vi "Merce Cmd.vi"() -> ()   [LabVIEW 2009]
panel:
  out "output Header":string[](array[string])
  out "Array":string[][](array[string])
  out "AMP":string[](array[string])
  out "FT":string[](array[string])
  out "RT":string[](array[string])
  out "WS1050 Cmd":string[](array[string])
  out "WS1050 Name":string[](array[string])
  in  "WS1050 C1L Cmd":string[](array[string])=["074101", "074100", "074102", "074100", "074104", "074108", "07410C", "074110", "074114", "074118", "07411C", "074120", "074124", "074128", "07412C", "074130", "074134", "074138", "074139", "07413B", "074139", "074138", "074134", "074130", "07412C", "074128", "074124", "074120", "07411C", "074118", "074114", "074110", "07410C", "074108", "074104", "074100", "", "", "", "", "", "", "", "", "", "", "", "", "", "", "", "", "", "", "", "", "", "", "", "", "", "", "", "", "", "", "", "", "", "", "", ""]
  in  "C1L":string[](array[string])=["C1L_S0F1_ON", "C1L_S0F1_OFF", "C1L_S0F2_ON", "C1L_S0F2_OFF", "C1L_S1_UP", "C1L_S2_UP", "C1L_S3_UP", "C1L_S4_UP", "C1L_S5_UP", "C1L_S6_UP", "C1L_S7_UP", "C1L_S8_UP", "C1L_S9_UP", "C1L_S10_UP", "C1L_S11_UP", "C1L_S12_UP", "C1L_S13_UP", "C1L_S14_UP", "C1L_S14F1_UP", "C1L_S14F12_UP", "C1L_S14F1_DN", "C1L_S14_DN", "C1L_S13_DN", "C1L_S12_DN", "C1L_S11_DN", "C1L_S10_DN", "C1L_S9_DN", "C1L_S8_DN", "C1L_S7_DN", "C1L_S6_DN", "C1L_S5_DN", "C1L_S4_DN", "C1L_S3_DN", "C1L_S2_DN", "C1L_S1_DN", "C1L_ALL_OFF"]
  in  "C3L":string[](array[string])=["C3L_S0F1_ON", "C3L_S0F1_OFF", "C3L_S0F2_ON", "C3L_S0F2_OFF", "C3L_S1_UP", "C3L_S2_UP", "C3L_S3_UP", "C3L_S4_UP", "C3L_S5_UP", "C3L_S6_UP", "C3L_S7_UP", "C3L_S8_UP", "C3L_S9_UP", "C3L_S10_UP", "C3L_S11_UP", "C3L_S12_UP", "C3L_S13_UP", "C3L_S14_UP", "C3L_S14F1_UP", "C3L_S14F12_UP", "C3L_S14F1_DN", "C3L_S14_DN", "C3L_S13_DN", "C3L_S12_DN", "C3L_S11_DN", "C3L_S10_DN", "C3L_S9_DN", "C3L_S8_DN", "C3L_S7_DN", "C3L_S6_DN", "C3L_S5_DN", "C3L_S4_DN", "C3L_S3_DN", "C3L_S2_DN", "C3L_S1_DN", "C3L_ALL_OFF"]
  in  "C2L":string[](array[string])=["C2L_S0F1_ON", "C2L_S0F1_OFF", "C2L_S0F2_ON", "C2L_S0F2_OFF", "C2L_S1_UP", "C2L_S2_UP", "C2L_S3_UP", "C2L_S4_UP", "C2L_S5_UP", "C2L_S6_UP", "C2L_S7_UP", "C2L_S8_UP", "C2L_S9_UP", "C2L_S10_UP", "C2L_S11_UP", "C2L_S12_UP", "C2L_S13_UP", "C2L_S14_UP", "C2L_S14F1_UP", "C2L_S14F12_UP", "C2L_S14F1_DN", "C2L_S14_DN", "C2L_S13_DN", "C2L_S12_DN", "C2L_S11_DN", "C2L_S10_DN", "C2L_S9_DN", "C2L_S8_DN", "C2L_S7_DN", "C2L_S6_DN", "C2L_S5_DN", "C2L_S4_DN", "C2L_S3_DN", "C2L_S2_DN", "C2L_S1_DN", "C2L_ALL_OFF"]
  in  "WS1050 C3L Cmd":string[](array[string])=["074301", "074300", "074302", "074300", "074304", "074308", "07430C", "074310", "074314", "074318", "07431C", "074320", "074324", "074328", "07432C", "074330", "074334", "074338", "074339", "07433B", "074339", "074338", "074334", "074330", "07432C", "074328", "074324", "074320", "07431C", "074318", "074314", "074310", "07430C", "074308", "074304", "074300"]
  in  "WS1050 C2L Cmd":string[](array[string])=["074201", "074200", "074202", "074200", "074204", "074208", "07420C", "074210", "074214", "074218", "07421C", "074220", "074224", "074228", "07422C", "074230", "074234", "074238", "074239", "07423B", "074239", "074238", "074234", "074230", "07422C", "074228", "074224", "074220", "07421C", "074218", "074214", "074210", "07420C", "074208", "074204", "074200"]
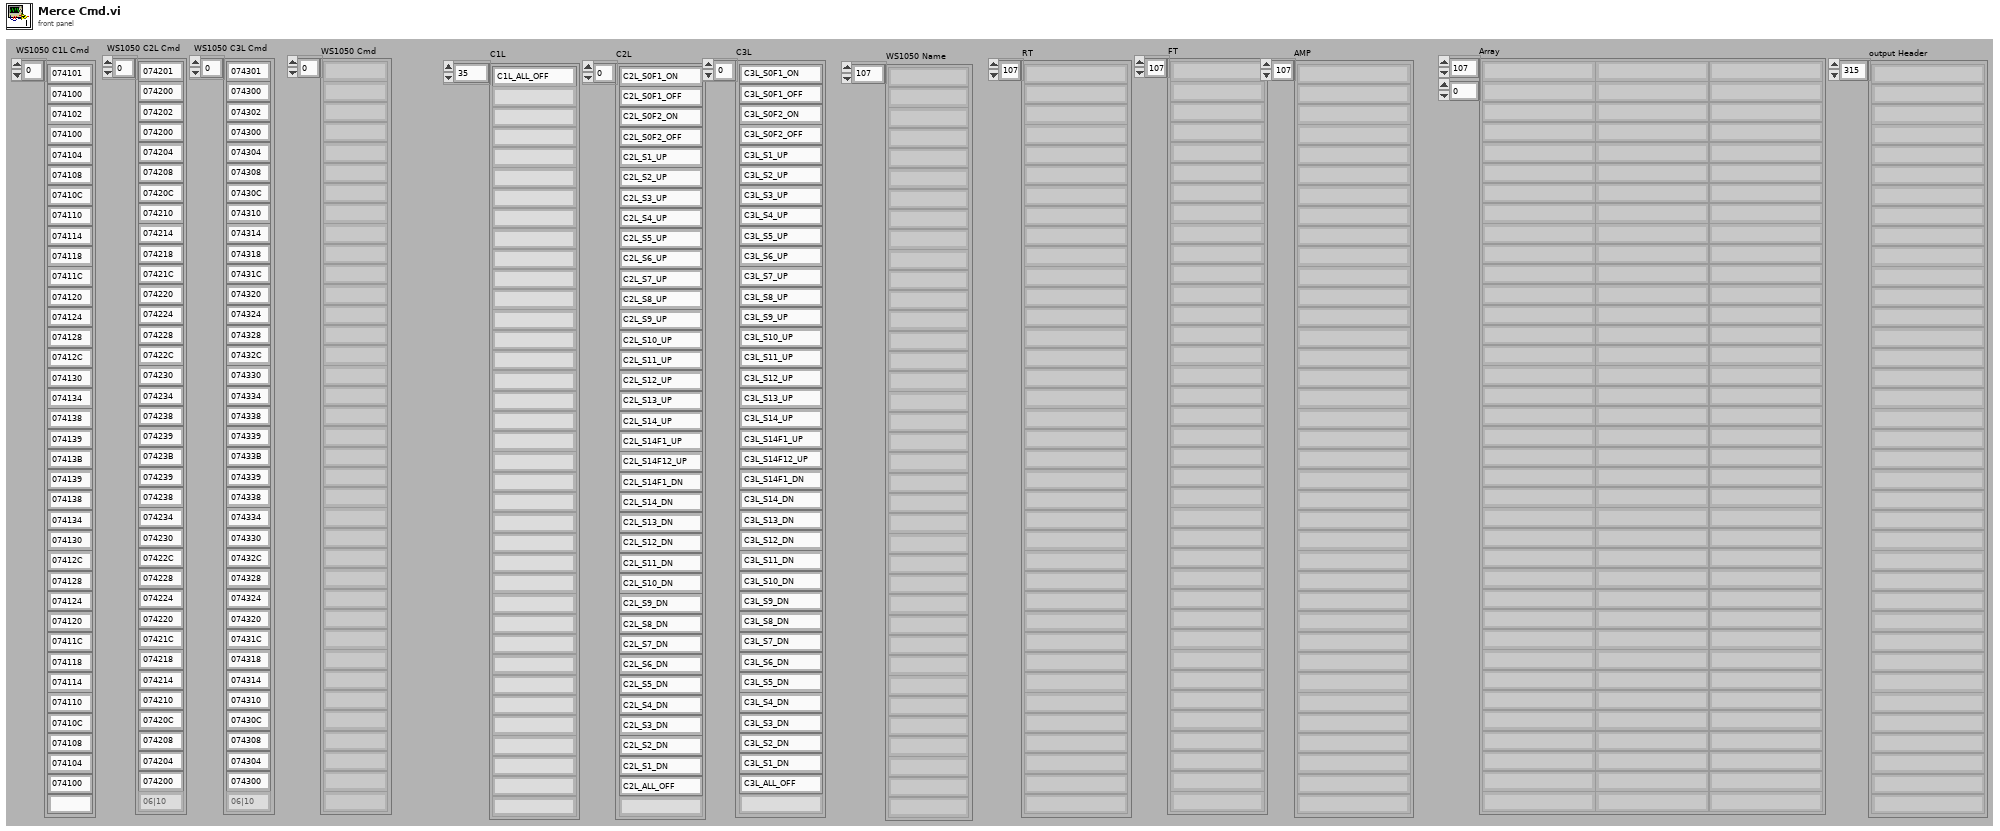
[diagram p1: front panel]
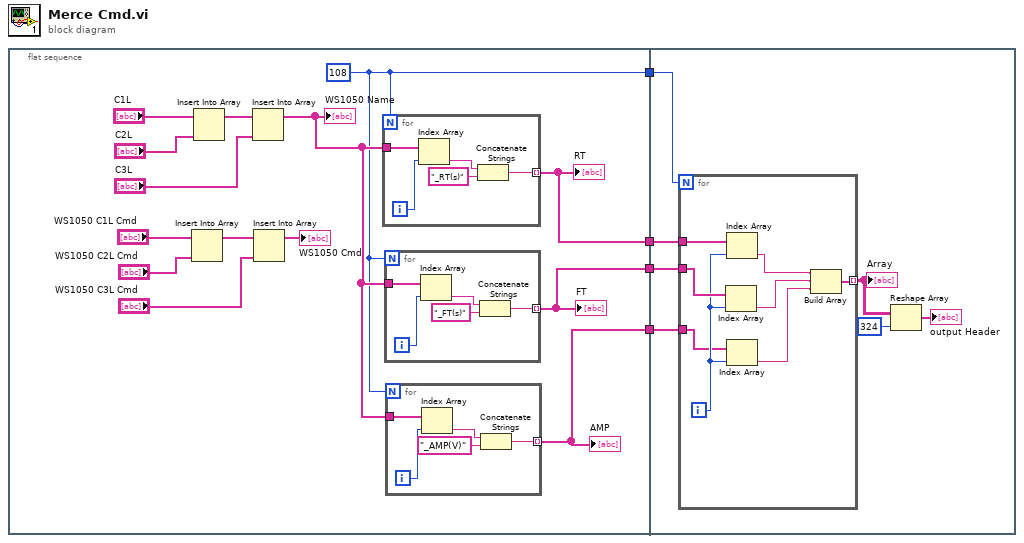
[diagram p0: block diagram]
diagram:
  n1 = flat-sequence {
    tunnel: [w8] -> w4
    tunnel: [w7] -> w3
    tunnel: [w6] -> w2
    tunnel: [w5] -> w1
    tunnel: w4 -> [w40]
    tunnel: w3 -> [w39]
    tunnel: w2 -> [w38]
    tunnel: w1 -> [w37]
    frame #0 {
      w5 = 108
      n2 = Insert Into Array(array="WS1050 C1L Cmd", new element="WS1050 C2L Cmd") -> (w14:string[])  [unwired: 1 in]
      n3 = Insert Into Array(array="C1L", new element="C2L") -> (w16:string[])  [unwired: 1 in]
      n4 = Insert Into Array(array=w16, new element="C3L") -> (w9:string[])  [unwired: 1 in]
      "WS1050 Name" <- w9
      n5 = Insert Into Array(array=w14, new element="WS1050 C3L Cmd") -> (→"WS1050 Cmd":string[])  [unwired: 1 in]
      n6 = for {
        N: w5 -> [_]
        tunnel: w9 -> [w33]
        tunnel: [w29] -> w7 mode=indexing
        i -> [w32]
        n7 = Index Array(array=w33, index=w32) -> (element=w31:string)
        n8 = Concatenate Strings(w31, "_RT(s)" ("string")) -> (w29:string)
      }
      "RT" <- w7
      n9 = for {
        N: w5 -> [_]
        tunnel: w9 -> [w28]
        tunnel: [w24] -> w8 mode=indexing
        i -> [w27]
        n10 = Index Array(array=w28, index=w27) -> (element=w26:string)
        n11 = Concatenate Strings(w26, "_FT(s)" ("string")) -> (w24:string)
      }
      "FT" <- w8
      n12 = for {
        N: w5 -> [_]
        tunnel: w9 -> [w23]
        tunnel: [w19] -> w6 mode=indexing
        i -> [w22]
        n13 = Index Array(array=w23, index=w22) -> (element=w21:string)
        n14 = Concatenate Strings(w21, "_AMP(V)" ("string")) -> (w19:string)
      }
      "AMP" <- w6
    }
    frame #1 {
      n15 = for {
        N: w37 -> [_]
        tunnel: w40 -> [w47]
        tunnel: w39 -> [w48]
        tunnel: w38 -> [w45]
        tunnel: [w41] -> w36 mode=indexing
        i -> [w46]
        n16 = Index Array(array=w47, index=w46) -> (element=w43:string)
        n17 = Index Array(array=w48, index=w46) -> (element=w44:string)
        n18 = Index Array(array=w45, index=w46) -> (element=w42:string)
        n19 = Build Array(w44, w43, w42) -> (w41:string[])
      }
      "Array" <- w36
      n20 = Reshape Array(w36, 324 ("dimension size")) -> (→"output Header":string[])
    }
  }
